vi "test Import To Empty Module Different Slot.vi"(8 "error in (no error)":errorcluster, 11 "TestCase in":refnum<class "NI-SWITCH Import Export Unit Tests.lvclass">) -> (0 "error out":errorcluster, 3 "TestCase out":refnum<class "NI-SWITCH Import Export Unit Tests.lvclass">)   [LabVIEW 2017, in "NI-SWITCH Import Export Unit Tests.lvclass"]
uses:
  NI-SWITCH Import Export Unit Tests.lvclass
  Shared/Endpoint Configuration Cluster.ctl
  Shared/Endpoint Configuration Enum.ctl
  NI-SWITCH Import Export Unit Tests.lvclass/NI-SWITCH Import Export Unit Tests.ctl
  <vilib>/NI Veristand/Custom Device API/Get Item Property (U32).vi
  <vilib>/addons/_JKI Toolkits/VI Tester/TestCase.llb/TestCase.lvclass
  <vilib>/NI/NI VeriStand Custom Device Import and Export Tool/ImportExport.lvlib
  Scripting/NI-SWITCH Scripting.lvlib
  Shared/VeriStand System Definition Test Utilities/VeriStand System Definition Test Utilities.lvlib
  Shared/NI-SWITCH Shared.lvlib
  <vilib>/NI VeriStand/Custom Device API/Custom Device API.lvlib
  C:/Program Files (x86)/National Instruments/LabVIEW 2017/vi.lib/addons/_JKI Toolkits/VI Tester/TestCase.llb/TestCase.lvclass
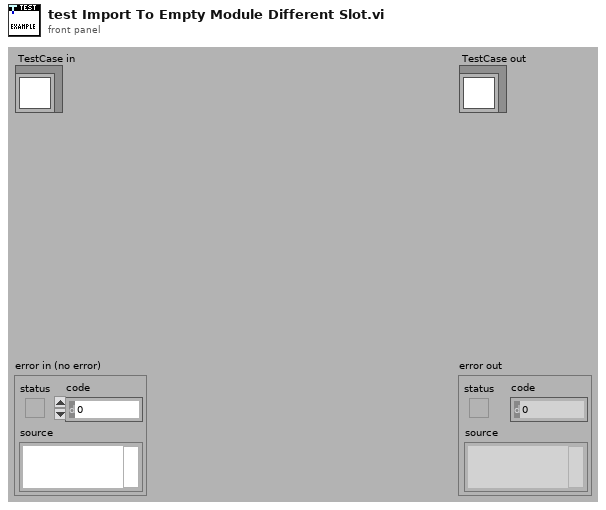
[diagram p1: front panel]
types:
  T1 = cluster{"Ignore Properties":string[], "Ignore Top Level Name":bool}
  T2 = typedef "NI-SWITCH Shared.lvlib/Endpoint Configuration Cluster.ctl" = cluster{"Endpoint":string, "Configuration":T3}
  T3 = typedef "NI-SWITCH Shared.lvlib/Endpoint Configuration Enum.ctl" = enum16{"Load", "Source", "Configuration"}
  T4 = typedef "Custom Device API.lvlib/Custom Device Item Ref.ctl" = u64
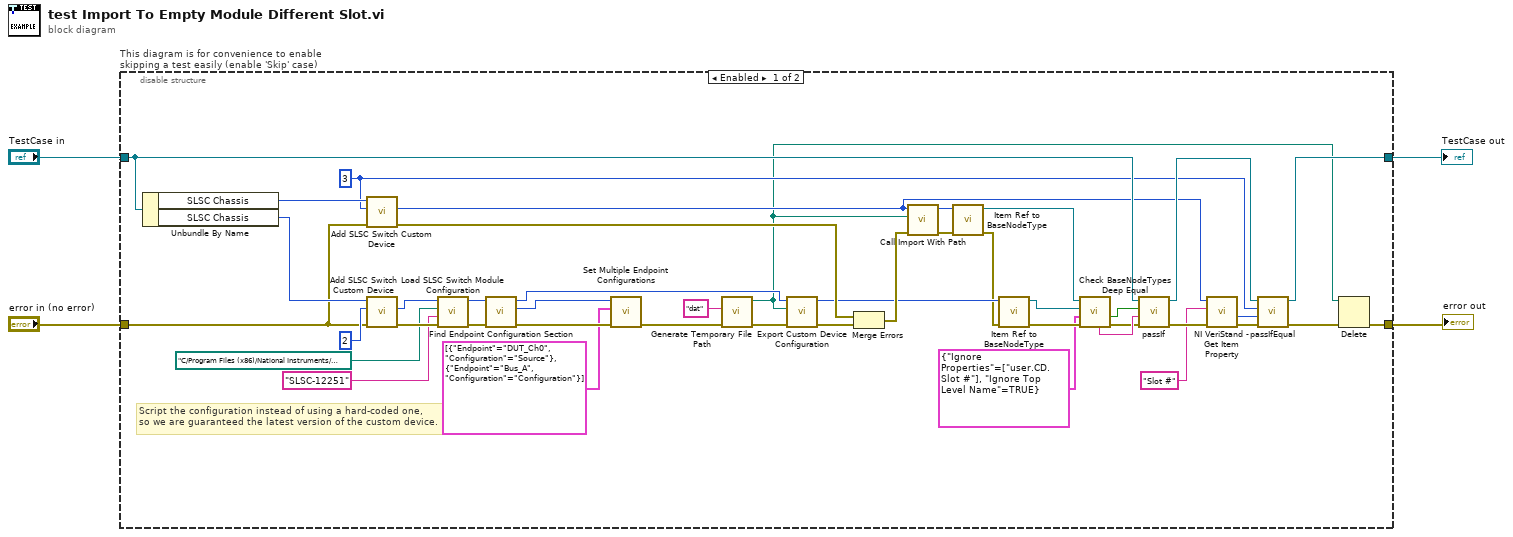
[diagram p0: block diagram]
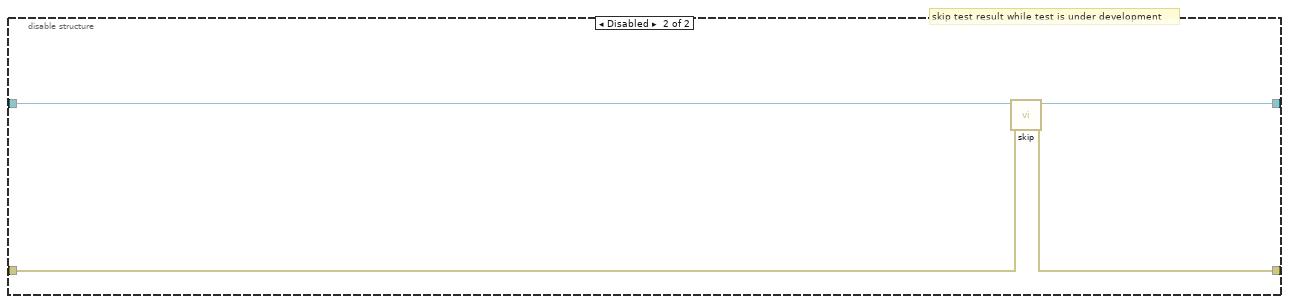
[diagram p2: hidden frame]
diagram:
  n1 = disable-structure "This diagram is for convenience to enable skipping a test easily (enable 'Skip' case)" shown="Enabled" {
    disable-tunnel: "TestCase in" -> [w33 w51]
    disable-tunnel: [w12 w49] -> w1
    disable-tunnel: [w6 w50] -> w3
    disable-tunnel: "error in (no error)" -> [w27 w48]
    frame Enabled {
      w9 = u32 3 ("slot number")
      # "Script the configuration instead of using a hard-coded one,\nso we are guaranteed the latest version of the custom device."
      n2 = Unbundle By Name(w33) -> ("SLSC Chassis"=w28:u64, "SLSC Chassis"=w47:u64)
      n3 = call "Add SLSC Switch Custom Device.vi"("error in"=w27, "slot number"=w9, "slsc chassis in"=w28) -> ("error out"=w42:errorcluster, "slsc switch custom device"=w8:T4)  [unwired: 6 in, 1 out]
      n4 = call "Add SLSC Switch Custom Device.vi"("error in"=w27, "slot number"=u32 2, "slsc chassis in"=w47) -> ("error out"=w26:errorcluster, "slsc switch custom device"=w24:T4)  [unwired: 6 in, 1 out]
      n5 = call "Load SLSC Switch Module Configuration.vi"("error in"=w26, "product name"="SLSC-12251", "switches json file"=path "C:/Program Files (x86)/National Instruments/Shared/NI-SLSC Switch/Modules/SLSC-12251-switches.json", "slsc switch custom device in"=w24) -> ("error out"=w25:errorcluster, "slsc switch custom device out"=w20:T4)  [unwired: 6 in]
      n6 = call "Find Endpoint Configuration Section.vi"("error in"=w25, "slsc switch custom device in"=w20) -> ("error out"=w21:errorcluster, "endpoint configuration"=w18:T4, "slsc switch custom device out"=w17:T4)  [unwired: 7 in]
      n7 = call "Set Multiple Endpoint Configurations.vi"("error in"=w21, "endpoint configurations"=T2[] [{"Endpoint"="DUT_Ch0", "Configuration"=enum."Source"}, {"Endpoint"="Bus_A", "Configuration"=enum."Configuration"}], "endpoint configuration in"=w18) -> ("error out"=w19:errorcluster)  [unwired: 7 in, 1 out]
      n8 = call <vilib>:"Generate Temporary File Path.vi"("error in (no error)"=w19, "Temporary File Extension (tmp)"="dat") -> ("error out"=w44:errorcluster, "Unique Temporary File Path"=w5:path)  [unwired: 8 in]
      n9 = call <vilib>:"Export Custom Device Configuration.vi"("error in (no error)"=w44, "Path"=w5, "ID"=w17) -> ("error out"=w43:errorcluster, "ID out"=w39:u64)  [unwired: 7 in]
      n10 = Merge Errors(w42, w43) -> (w41:errorcluster)
      n11 = call "Call Import With Path.vi"("error in (no error)"=w41, "Path"=w5, "Node Ptr"=w8) -> ("error out"=w38:errorcluster, "Node Ptr out"=w40:u64)  [unwired: 7 in]
      n12 = call "Item Ref to BaseNodeType.vi"("error in (no error)"=w38, "Item Ref"=w40) -> ("error out"=w37:errorcluster, "BaseNodeType"=w30:refnum<k24>)  [unwired: 8 in]
      n13 = call "Item Ref to BaseNodeType.vi"("error in (no error)"=w37, "Item Ref"=w39) -> ("error out"=w36:errorcluster, "BaseNodeType"=w35:refnum<k24>)  [unwired: 8 in]
      n14 = call "Check BaseNodeTypes Deep Equal.vi"("error in (no error)"=w36, "Settings"=T1 {"Ignore Properties"=["user.CD.Slot #"], "Ignore Top Level Name"=TRUE}, "BaseNodeType 2"=w35, "BaseNodeType 1"=w30) -> ("error out"=w29:errorcluster, "Equal?"=w32:bool, "Inequality context"=w31:string)  [unwired: 3 in, 2 out]
      n15 = call-dynamic "passIf.vi"("error in (no error)"=w29, "message (\"\")"=w31, "pass"=w32, "TestCase in"=w33) -> ("error out"=w34:errorcluster, "TestCase out"=w13:refnum<class "NI-SWITCH Import Export Unit Tests.lvclass">)  [unwired: 6 in]
      n16 = call-poly <vilib>:"NI VeriStand - Get Item Property.vi"("error in (no error)"=w34, "Property Name"="Slot #", "Item Ref in"=w8) -> ("error out"=w11:errorcluster, "Value"=w10:u32)  [unwired: 5 in, 2 out]
      n17 = call-dynamic "passIfEqual.vi"("error in (no error)"=w11, "y"=w10, "x"=w9, "TestCase in"=w13) -> ("error out"=w14:errorcluster, "TestCase out"=w12:refnum<class "NI-SWITCH Import Export Unit Tests.lvclass">)  [unwired: 6 in]
      n18 = Delete(path (use dialog)=w5, error in=w14) -> (error out=w6:errorcluster)  [unwired: 3 in, 2 out]
    }
    frame Disabled {
      # "skip test result while test is under development"
      n19 = call <vilib>:"skip.vi"("error in (no error)"=w48, "TestCase in"=w51) -> ("error out"=w50:errorcluster, "TestCase out"=w49:refnum<class "NI-SWITCH Import Export Unit Tests.lvclass">)  [unwired: 8 in]
    }
  }
  "error out" <- w3
  "TestCase out" <- w1
